vi "Stop Appender by ID.vi"(8 "error in (no error)":errorcluster, 10 "id":string, 11 "Logger in":refnum<class "Logger.lvclass">) -> (0 "error out":errorcluster, 2 "found":bool, 3 "Logger out":refnum<class "Logger.lvclass">)   [LabVIEW 2026, in "Tests.lvlib"]
doc: "Test-support Act step: stops one registered appender's actor to simulate a stop/error fault (SRS-LMBR-021), while leaving it in the manager registry so the manager still broadcasts to the now-dead enqueuer.\nReads the current Snapshot via Logger's community Get Current Snapshot accessor, finds the RegistryEntry whose id matches id in, and sends Actor Framework Normal Stop to that entry's Message Enqueuer. Guarded on error in (passes through as a no-op). Does not unregister (that is UnregisterAppender / T-032); the registry entry stays so fault isolation can be observed.\nTests.lvlib, friend of Lumberjack.lvlib. Not a test."
uses:
  Tests.lvlib
  src/Public/Logger.lvclass/Logger.lvclass
  <vilib>/ActorFramework/Message Enqueuer/Message Enqueuer.lvclass/Message Enqueuer.ctl
  <vilib>/ActorFramework/Message Enqueuer/Enqueue.vi
  <vilib>/ActorFramework/Stop Msg/Stop Msg.lvclass
  <vilib>/ActorFramework/Message Priority Queue/Priority Enqueue.vi
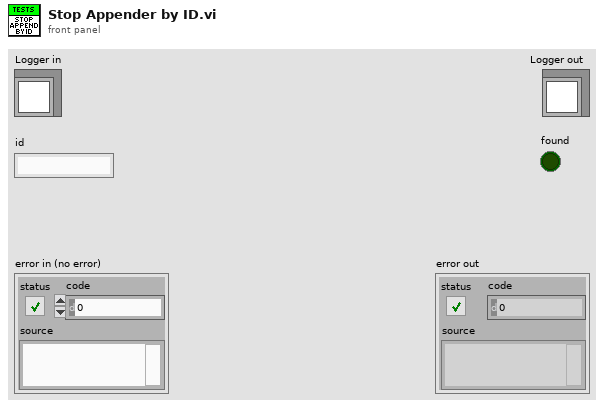
[diagram p1: front panel]
types:
  T1 = typedef "Lumberjack.lvlib/Snapshot.ctl" = cluster{"globalThreshold":T2, "appenders":cluster{"id":string, "enqueuer":refnum<class "Message Enqueuer.lvclass">}[]}
  T2 = typedef "Lumberjack.lvlib/Severity.ctl" = enum16{"OFF", "FATAL", "ERROR", "WARN", "INFO", "DEBUG", "TRACE", "ALL"}
  T3 = cluster{"id":string, "enqueuer":refnum<class "Message Enqueuer.lvclass">}[]
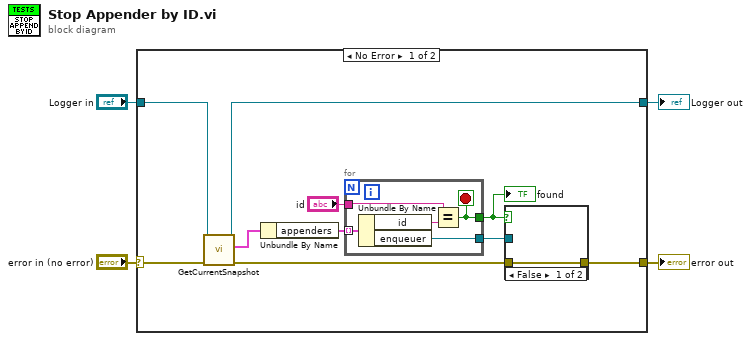
[diagram p0: block diagram]
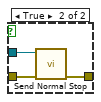
[diagram p2: hidden frame]
diagram:
  n1 = case shown="No Error" "error in (no error)" {
    selector: "error in (no error)" -> [w5 w25]
    tunnel: "Logger in" -> [w13 w24]
    tunnel: [w12 w24] -> w3
    tunnel: [w7 w25] -> w2
    frame No Error {
      n2 = call "GetCurrentSnapshot.vi"("error in (no error)"=w5, "Logger in"=w13) -> ("error out"=w8:errorcluster, "Snapshot"=w14:T1, "Logger out"=w12:refnum<class "Logger.lvclass">)  [unwired: 7 in]
      n3 = Unbundle By Name(w14) -> ("appenders"=w11:T3)
      n4 = for {
        tunnel: w11 -> [w23] mode=indexing
        tunnel: "id" -> [w22]
        tunnel: [w20] -> w6
        tunnel: [w19] -> w9
        stop <- w20 stop-if-true
        n5 = Unbundle By Name(w23) -> ("id"=w21:string, "enqueuer"=w19:refnum<class "Message Enqueuer.lvclass">)
        n6 = Equal?(x=w22, y=w21) -> (x = y?=w20:bool)
      }
      "found" <- w6
      n7 = case shown="False" w6 {
        tunnel: w9 -> [_ w18]
        tunnel: w8 -> [w15 w17]
        tunnel: [w15 w16] -> w7
        frame False {
        }
        frame True {
          n8 = call <vilib>:"Send Normal Stop.vi"("error in (no error)"=w17, "Message Enqueuer"=w18) -> ("error out"=w16:errorcluster)  [unwired: 9 in]
        }
      }
    }
    frame Error {
    }
  }
  "error out" <- w2
  "Logger out" <- w3
